vi "Untitled 2.vi"(8 "error in (no error)":errorcluster, 11 "Class 1 in":refnum<class "Class 1.lvclass">) -> (0 "error out":errorcluster, 2 "Numeric":dbl, 3 "Class 1 out":refnum<class "Class 1.lvclass">)   [LabVIEW 2023, in "Class 1.lvclass"]
uses:
  Class 1.lvclass
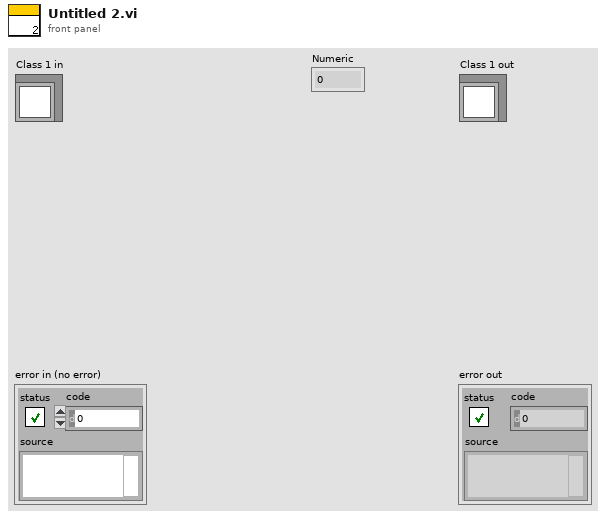
[diagram p1: front panel]
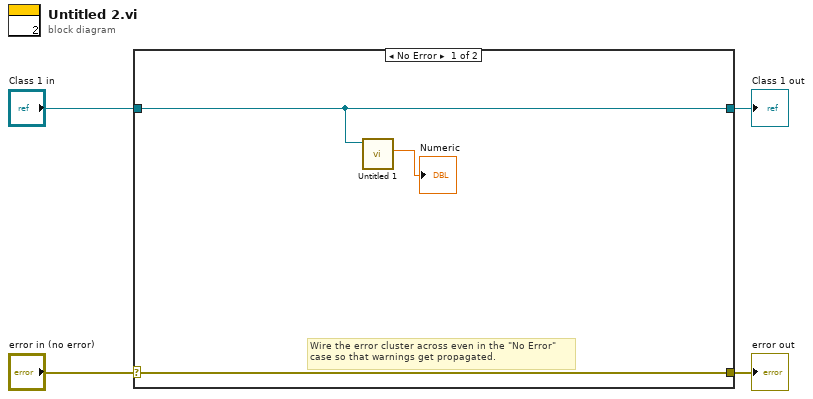
[diagram p0: block diagram]
diagram:
  n1 = case shown="No Error" "error in (no error)" {
    selector: "error in (no error)" -> [w7 w9]
    tunnel: [w7 w9] -> w3
    tunnel: [w5 w8] -> w1
    tunnel: "Class 1 in" -> [w5 w8]
    frame No Error {
      # "Wire the error cluster across even in the \"No Error\"\ncase so that warnings get propagated."
      n2 = call-dynamic "Untitled 1.vi"("Class 1 in"=w5) -> ("Numeric"=→"Numeric":dbl)  [unwired: 8 in, 2 out]
    }
    frame Error {
    }
  }
  "error out" <- w3
  "Class 1 out" <- w1
